vi "Guys Version_Acquire Pack and Push.vi"(9 "FIFO Refs":T1={"FIFO 0"="Simulation FIFO 0", "FIFO 1"="Simulation FIFO 1", "FIFO 2"="Simulation FIFO 2", "FIFO 3"="Simulation FIFO 3", "FIFO 4"="Simulation FIFO 4", "FIFO 5"="Simulation FIFO 5"}, 11 "Input Valid":bool) -> (3 "Ready for Input":bool)   [LabVIEW 2014]
uses:
  FPGA_Controls/Acquisition FIFOs Cluster.ctl
  <vilib>/rvi/eio/common/nirviEmuTemplateMethod_errors.vi
  <vilib>/rvi/DataTransferAndStorage/Container/Common/niFpgaContainerExecOnDevCompGetState.vi
  <vilib>/rvi/Emulation/niFpgaEmulationIsFPGAContextNoSignature.vi
  <vilib>/rvi/Emulation/niFpgaSctlEmulationGetInTimedLoop.vi
  <vilib>/rvi/errors/niFpgaSetErrorForExecOnDevCompSimple.vi
  <vilib>/rvi/eio/common/nirviEmuReportErrorAndStop.vi
  <vilib>/rvi/DataTransferAndStorage/Container/Common/niFpgaContainerGetUniqueNameForEmu.vi
  <vilib>/rvi/FIFO/Fifo_Resource/nirvififoEmulationSetSize.vi
  <vilib>/rvi/FIFO/Fifo_Resource/nirviFifoEmulationQueueMgr.vi
  <instcachedir>/0/nirviFifoEmulationQueueMgr_E5CAEC123FF24DC58D834DCA3CDAA9B5.lvgen/nirviFifoEmulationQueueMgr_E5CAEC123FF24DC58D834DCA3CDAA9B5_016.vi
  <vilib>/rvi/FIFO/Fifo_Resource/nirvififoEmulationDetermineInputValidOut.vi
  <vilib>/rvi/FIFO/Fifo_Resource/nirvififoEmulationCreateLock.vi
  <vilib>/rvi/Emulation/niFpgaProcessEmulError.vi
  <vilib>/rvi/FIFO/Fifo_Resource/nirvififoEmulationObtainLock.vi
  <vilib>/rvi/FIFO/Fifo_Resource/nirvififoEmulationReleaseLock.vi
  <vilib>/rvi/occurrence/nirviWaitOnOccurrenceBase.vi
  <vilib>/rvi/errors/nirviReportUnexpectedCaseInternalError.vi
  <vilib>/rvi/errors/nirviReportUnexpectedCaseInternalError (U32).vi
  <vilib>/rvi/interface/RandomDataEmulation/niFpgaRandomDataHandleErrors.vi
  <vilib>/eio/EIONode/EIONode.xnode
  <vilib>/rvi/DataTransferAndStorage/Container/XNode/niFpgaContainer.xnode
  <vilib>/rvi/FIFO/Fifo_Resource/niFpgaFifoEmulationRefIn.vi
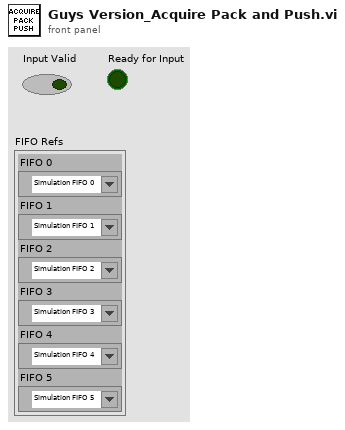
[diagram p1: front panel]
types:
  T1 = typedef "Acquisition FIFOs Cluster.ctl" = cluster{"FIFO 0":refnum<k21>, "FIFO 1":refnum<k21>, "FIFO 2":refnum<k21>, "FIFO 3":refnum<k21>, "FIFO 4":refnum<k21>, "FIFO 5":refnum<k21>}
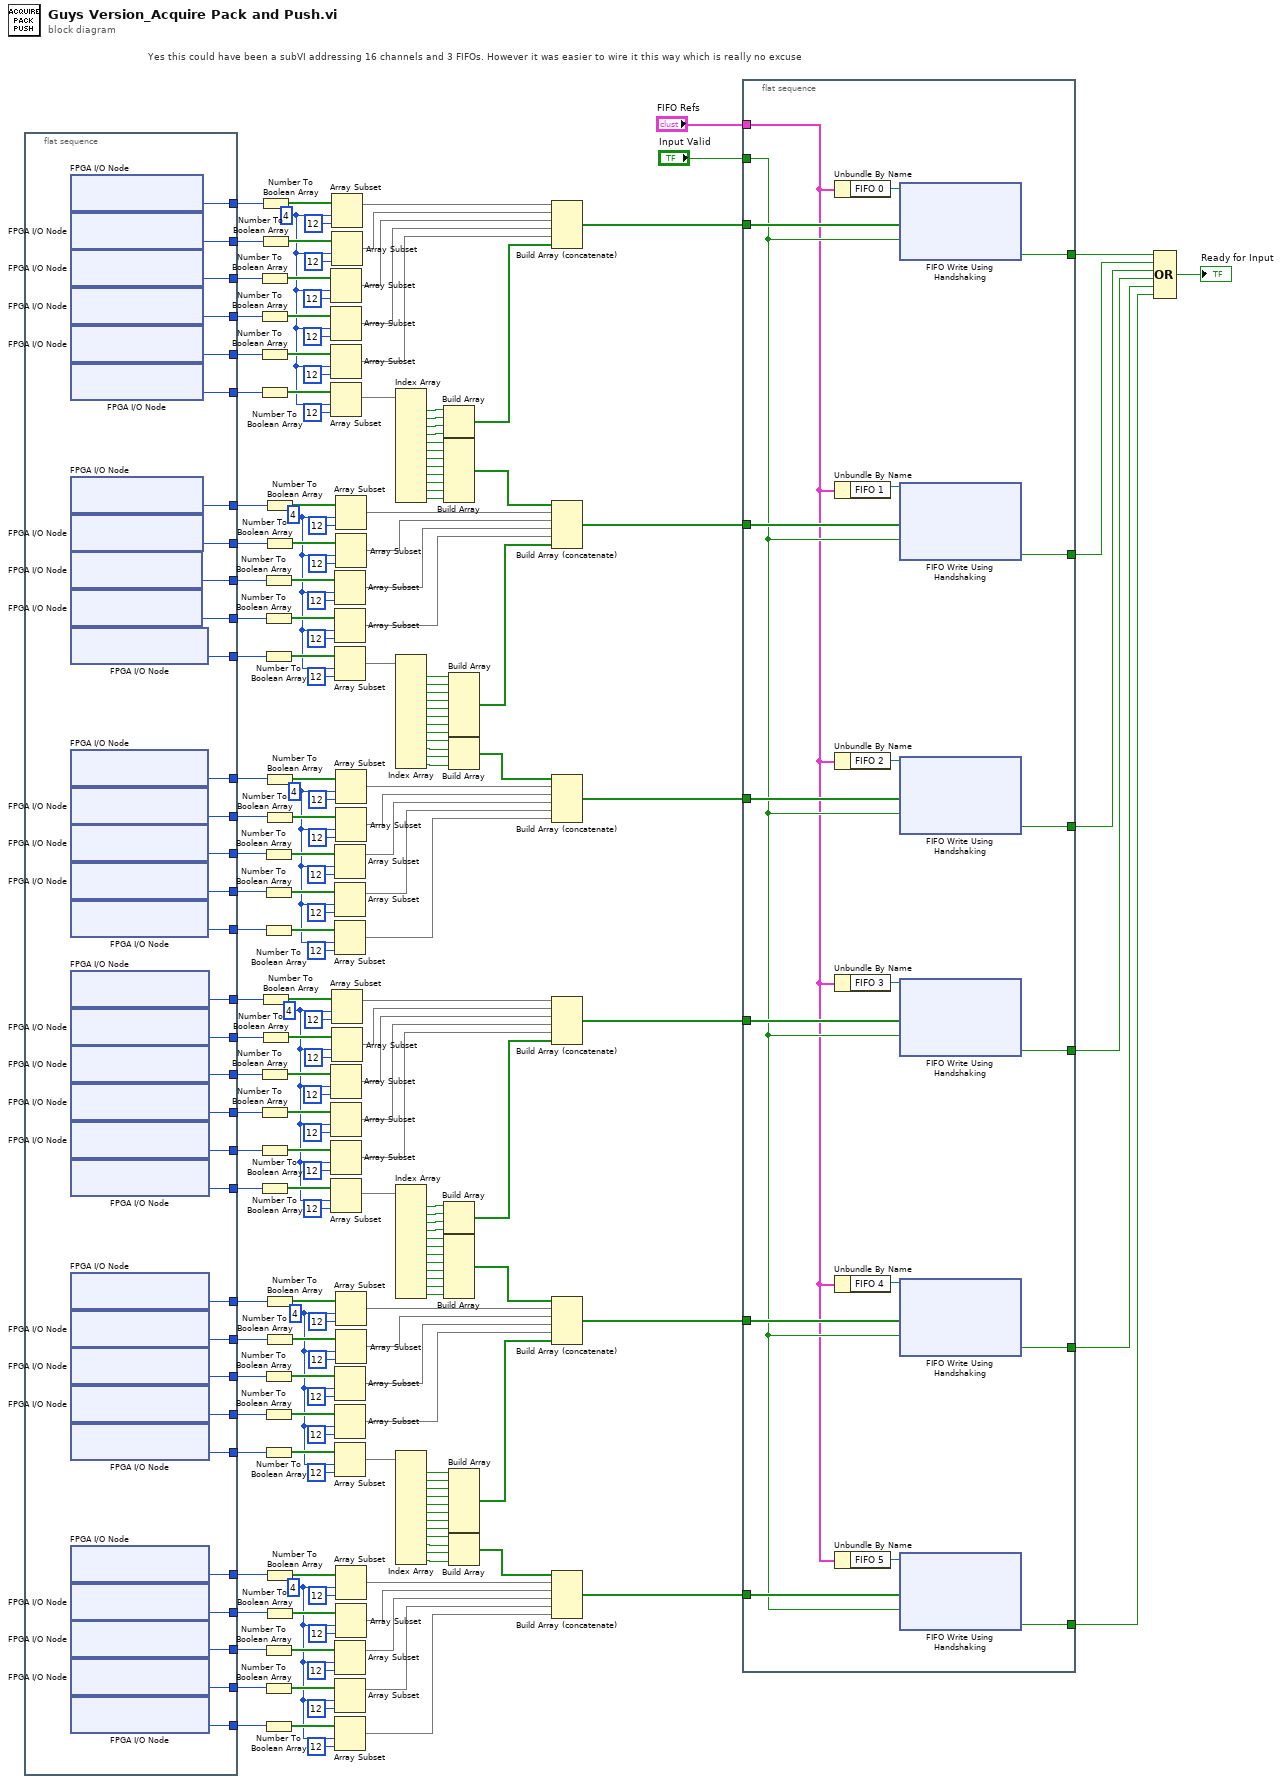
[diagram p0: block diagram]
diagram:
  w1 = 4 ("length")
  w2 = 4 ("index")
  w3 = 4 ("index")
  w4 = 4 ("index")
  w5 = 4 ("index")
  w6 = 4 ("index")
  # "Yes this could have been a subVI addressing 16 channels and 3 FIFOs. However it was easier to wire it this way which is really no excuse"
  n1 = flat-sequence {
    tunnel: [w237] -> w86
    tunnel: [w236] -> w87
    tunnel: [w235] -> w88
    tunnel: [w234] -> w89
    tunnel: [w233] -> w90
    tunnel: [w232] -> w91
    tunnel: [w231] -> w92
    tunnel: [w230] -> w93
    tunnel: [w229] -> w94
    tunnel: [w228] -> w95
    tunnel: [w227] -> w96
    tunnel: [w226] -> w97
    tunnel: [w225] -> w98
    tunnel: [w224] -> w99
    tunnel: [w223] -> w100
    tunnel: [w222] -> w101
    tunnel: [w221] -> w108
    tunnel: [w220] -> w109
    tunnel: [w219] -> w110
    tunnel: [w218] -> w111
    tunnel: [w217] -> w112
    tunnel: [w216] -> w113
    tunnel: [w215] -> w114
    tunnel: [w214] -> w115
    tunnel: [w213] -> w116
    tunnel: [w212] -> w117
    tunnel: [w211] -> w118
    tunnel: [w210] -> w119
    tunnel: [w209] -> w120
    tunnel: [w208] -> w121
    tunnel: [w207] -> w122
    tunnel: [w206] -> w123
    frame #0 {
      n2 = xnode "FPGA I/O Node"() -> ("IO Module\\AI A0"=w237:i16)  [unwired: 1 in, 1 out]
      n3 = xnode "FPGA I/O Node"() -> ("IO Module\\AI A1"=w236:i16)  [unwired: 1 in, 1 out]
      n4 = xnode "FPGA I/O Node"() -> ("IO Module\\AI A2"=w235:i16)  [unwired: 1 in, 1 out]
      n5 = xnode "FPGA I/O Node"() -> ("IO Module\\AI A3"=w234:i16)  [unwired: 1 in, 1 out]
      n6 = xnode "FPGA I/O Node"() -> ("IO Module\\AI A4"=w233:i16)  [unwired: 1 in, 1 out]
      n7 = xnode "FPGA I/O Node"() -> ("IO Module\\AI A5"=w232:i16)  [unwired: 1 in, 1 out]
      n8 = xnode "FPGA I/O Node"() -> ("IO Module\\AI A6"=w231:i16)  [unwired: 1 in, 1 out]
      n9 = xnode "FPGA I/O Node"() -> ("IO Module\\AI A7"=w230:i16)  [unwired: 1 in, 1 out]
      n10 = xnode "FPGA I/O Node"() -> ("IO Module\\AI B8"=w229:i16)  [unwired: 1 in, 1 out]
      n11 = xnode "FPGA I/O Node"() -> ("IO Module\\AI B9"=w228:i16)  [unwired: 1 in, 1 out]
      n12 = xnode "FPGA I/O Node"() -> ("IO Module\\AI B10"=w227:i16)  [unwired: 1 in, 1 out]
      n13 = xnode "FPGA I/O Node"() -> ("IO Module\\AI B11"=w226:i16)  [unwired: 1 in, 1 out]
      n14 = xnode "FPGA I/O Node"() -> ("IO Module\\AI B12"=w225:i16)  [unwired: 1 in, 1 out]
      n15 = xnode "FPGA I/O Node"() -> ("IO Module\\AI B13"=w224:i16)  [unwired: 1 in, 1 out]
      n16 = xnode "FPGA I/O Node"() -> ("IO Module\\AI B14"=w223:i16)  [unwired: 1 in, 1 out]
      n17 = xnode "FPGA I/O Node"() -> ("IO Module\\AI B15"=w222:i16)  [unwired: 1 in, 1 out]
      n18 = xnode "FPGA I/O Node"() -> ("IO Module\\AI C16"=w206:i16)  [unwired: 1 in, 1 out]
      n19 = xnode "FPGA I/O Node"() -> ("IO Module\\AI C17"=w207:i16)  [unwired: 1 in, 1 out]
      n20 = xnode "FPGA I/O Node"() -> ("IO Module\\AI C18"=w208:i16)  [unwired: 1 in, 1 out]
      n21 = xnode "FPGA I/O Node"() -> ("IO Module\\AI C19"=w209:i16)  [unwired: 1 in, 1 out]
      n22 = xnode "FPGA I/O Node"() -> ("IO Module\\AI C20"=w210:i16)  [unwired: 1 in, 1 out]
      n23 = xnode "FPGA I/O Node"() -> ("IO Module\\AI C21"=w211:i16)  [unwired: 1 in, 1 out]
      n24 = xnode "FPGA I/O Node"() -> ("IO Module\\AI C22"=w212:i16)  [unwired: 1 in, 1 out]
      n25 = xnode "FPGA I/O Node"() -> ("IO Module\\AI C23"=w213:i16)  [unwired: 1 in, 1 out]
      n26 = xnode "FPGA I/O Node"() -> ("IO Module\\AI D24"=w214:i16)  [unwired: 1 in, 1 out]
      n27 = xnode "FPGA I/O Node"() -> ("IO Module\\AI D25"=w215:i16)  [unwired: 1 in, 1 out]
      n28 = xnode "FPGA I/O Node"() -> ("IO Module\\AI D26"=w216:i16)  [unwired: 1 in, 1 out]
      n29 = xnode "FPGA I/O Node"() -> ("IO Module\\AI D27"=w217:i16)  [unwired: 1 in, 1 out]
      n30 = xnode "FPGA I/O Node"() -> ("IO Module\\AI D28"=w218:i16)  [unwired: 1 in, 1 out]
      n31 = xnode "FPGA I/O Node"() -> ("IO Module\\AI D29"=w219:i16)  [unwired: 1 in, 1 out]
      n32 = xnode "FPGA I/O Node"() -> ("IO Module\\AI D30"=w220:i16)  [unwired: 1 in, 1 out]
      n33 = xnode "FPGA I/O Node"() -> ("IO Module\\AI D31"=w221:i16)  [unwired: 1 in, 1 out]
    }
  }
  n34 = Number To Boolean Array(number=w88) -> (Boolean array=w19:bool[])
  n35 = Number To Boolean Array(number=w89) -> (Boolean array=w16:bool[])
  n36 = Number To Boolean Array(number=w90) -> (Boolean array=w25:bool[])
  n37 = Number To Boolean Array(number=w91) -> (Boolean array=w22:bool[])
  n38 = Number To Boolean Array(number=w121) -> (Boolean array=w190:bool[])
  n39 = Number To Boolean Array(number=w120) -> (Boolean array=w193:bool[])
  n40 = Number To Boolean Array(number=w119) -> (Boolean array=w184:bool[])
  n41 = Number To Boolean Array(number=w118) -> (Boolean array=w187:bool[])
  n42 = Number To Boolean Array(number=w86) -> (Boolean array=w10:bool[])
  n43 = Number To Boolean Array(number=w87) -> (Boolean array=w13:bool[])
  n44 = Number To Boolean Array(number=w123) -> (Boolean array=w199:bool[])
  n45 = Number To Boolean Array(number=w122) -> (Boolean array=w196:bool[])
  n46 = Number To Boolean Array(number=w94) -> (Boolean array=w43:bool[])
  n47 = Number To Boolean Array(number=w95) -> (Boolean array=w46:bool[])
  n48 = Number To Boolean Array(number=w96) -> (Boolean array=w41:bool[])
  n49 = Number To Boolean Array(number=w99) -> (Boolean array=w77:bool[])
  n50 = Number To Boolean Array(number=w100) -> (Boolean array=w74:bool[])
  n51 = Number To Boolean Array(number=w101) -> (Boolean array=w79:bool[])
  n52 = Number To Boolean Array(number=w115) -> (Boolean array=w166:bool[])
  n53 = Number To Boolean Array(number=w114) -> (Boolean array=w163:bool[])
  n54 = Number To Boolean Array(number=w113) -> (Boolean array=w168:bool[])
  n55 = Number To Boolean Array(number=w110) -> (Boolean array=w132:bool[])
  n56 = Number To Boolean Array(number=w109) -> (Boolean array=w135:bool[])
  n57 = Number To Boolean Array(number=w108) -> (Boolean array=w130:bool[])
  n58 = Number To Boolean Array(number=w92) -> (Boolean array=w50:bool[])
  n59 = Number To Boolean Array(number=w93) -> (Boolean array=w47:bool[])
  n60 = Number To Boolean Array(number=w97) -> (Boolean array=w70:bool[])
  n61 = Number To Boolean Array(number=w98) -> (Boolean array=w73:bool[])
  n62 = Number To Boolean Array(number=w117) -> (Boolean array=w159:bool[])
  n63 = Number To Boolean Array(number=w116) -> (Boolean array=w162:bool[])
  n64 = Number To Boolean Array(number=w112) -> (Boolean array=w139:bool[])
  n65 = Number To Boolean Array(number=w111) -> (Boolean array=w136:bool[])
  n66 = Array Subset(array=w19, index=w6, length=12) -> (w20:bool[])
  n67 = Array Subset(array=w16, index=w6, length=12) -> (w21:bool[])
  n68 = Array Subset(array=w25, index=w6, length=12) -> (w26:bool[])
  n69 = Array Subset(array=w22, index=w6, length=12) -> (w27:bool[])
  n70 = Array Subset(array=w190, index=w3, length=12) -> (w189:bool[])
  n71 = Array Subset(array=w193, index=w3, length=12) -> (w188:bool[])
  n72 = Array Subset(array=w184, index=w3, length=12) -> (w183:bool[])
  n73 = Array Subset(array=w187, index=w3, length=12) -> (w182:bool[])
  n74 = Array Subset(array=w10, index=w6, length=12) -> (w14:bool[])
  n75 = Array Subset(array=w13, index=w6, length=12) -> (w15:bool[])
  n76 = Array Subset(array=w199, index=w3, length=12) -> (w195:bool[])
  n77 = Array Subset(array=w196, index=w3, length=12) -> (w194:bool[])
  n78 = Array Subset(array=w43, index=w5, length=12) -> (w54:bool[])
  n79 = Array Subset(array=w46, index=w5, length=12) -> (w55:bool[])
  n80 = Array Subset(array=w41, index=w5, length=12) -> (w56:bool[])
  n81 = Array Subset(array=w77, index=w4, length=12) -> (w83:bool[])
  n82 = Array Subset(array=w74, index=w4, length=12) -> (w84:bool[])
  n83 = Array Subset(array=w79, index=w4, length=12) -> (w85:bool[])
  n84 = Array Subset(array=w166, index=w2, length=12) -> (w155:bool[])
  n85 = Array Subset(array=w163, index=w2, length=12) -> (w154:bool[])
  n86 = Array Subset(array=w168, index=w2, length=12) -> (w153:bool[])
  n87 = Array Subset(array=w132, index=w1, length=12) -> (w126:bool[])
  n88 = Array Subset(array=w135, index=w1, length=12) -> (w125:bool[])
  n89 = Array Subset(array=w130, index=w1, length=12) -> (w124:bool[])
  n90 = Array Subset(array=w50, index=w5, length=12) -> (w52:bool[])
  n91 = Array Subset(array=w47, index=w5, length=12) -> (w53:bool[])
  n92 = Array Subset(array=w70, index=w4, length=12) -> (w81:bool[])
  n93 = Array Subset(array=w73, index=w4, length=12) -> (w82:bool[])
  n94 = Array Subset(array=w159, index=w2, length=12) -> (w157:bool[])
  n95 = Array Subset(array=w162, index=w2, length=12) -> (w156:bool[])
  n96 = Array Subset(array=w139, index=w1, length=12) -> (w128:bool[])
  n97 = Array Subset(array=w136, index=w1, length=12) -> (w127:bool[])
  n98 = Index Array(array=w27) -> (element #1=w28:bool, element #2=w29:bool, element #3=w30:bool, element #4=w31:bool, element #5=w33:bool, element #6=w34:bool, element #7=w35:bool, element #8=w36:bool, element #9=w37:bool, element #10=w38:bool, element #11=w39:bool, element #12=w40:bool)  [unwired: 12 in]
  n99 = Index Array(array=w56) -> (element #1=w57:bool, element #2=w58:bool, element #3=w59:bool, element #4=w60:bool, element #5=w61:bool, element #6=w62:bool, element #7=w63:bool, element #8=w64:bool, element #9=w66:bool, element #10=w67:bool, element #11=w68:bool, element #12=w69:bool)  [unwired: 12 in]
  n100 = Index Array(array=w182) -> (element #1=w181:bool, element #2=w180:bool, element #3=w179:bool, element #4=w178:bool, element #5=w176:bool, element #6=w175:bool, element #7=w174:bool, element #8=w173:bool, element #9=w172:bool, element #10=w171:bool, element #11=w170:bool, element #12=w169:bool)  [unwired: 12 in]
  n101 = Index Array(array=w153) -> (element #1=w152:bool, element #2=w151:bool, element #3=w150:bool, element #4=w149:bool, element #5=w148:bool, element #6=w147:bool, element #7=w146:bool, element #8=w145:bool, element #9=w143:bool, element #10=w142:bool, element #11=w141:bool, element #12=w140:bool)  [unwired: 12 in]
  n102 = Build Array(w28, w29, w30, w31) -> (w32:bool[])
  n103 = Build Array(w33, w34, w35, w36, w37, w38, w39, w40) -> (w51:bool[])
  n104 = Build Array(w181, w180, w179, w178) -> (w177:bool[])
  n105 = Build Array(w176, w175, w174, w173, w172, w171, w170, w169) -> (w158:bool[])
  n106 = Build Array(w57, w58, w59, w60, w61, w62, w63, w64) -> (w65:bool[])
  n107 = Build Array(w66, w67, w68, w69) -> (w80:bool[])
  n108 = Build Array(w152, w151, w150, w149, w148, w147, w146, w145) -> (w144:bool[])
  n109 = Build Array(w143, w142, w141, w140) -> (w129:bool[])
  n110 = Build Array (concatenate)(w14, w15, w20, w21, w26, w32) -> (w102:bool[])
  n111 = Build Array (concatenate)(w51, w52, w53, w54, w55, w65) -> (w103:bool[])
  n112 = Build Array (concatenate)(w80, w81, w82, w83, w84, w85) -> (w104:bool[])
  n113 = Build Array (concatenate)(w195, w194, w189, w188, w183, w177) -> (w107:bool[])
  n114 = Build Array (concatenate)(w158, w157, w156, w155, w154, w144) -> (w106:bool[])
  n115 = Build Array (concatenate)(w129, w128, w127, w126, w125, w124) -> (w105:bool[])
  n116 = flat-sequence {
    tunnel: w102 -> [w257]
    tunnel: w103 -> [w256]
    tunnel: w104 -> [w255]
    tunnel: w105 -> [w254]
    tunnel: w106 -> [w253]
    tunnel: w107 -> [w252]
    tunnel: [w251] -> w200
    tunnel: [w250] -> w201
    tunnel: [w249] -> w202
    tunnel: [w248] -> w203
    tunnel: [w247] -> w204
    tunnel: [w246] -> w205
    tunnel: "Input Valid" -> [w245]
    tunnel: "FIFO Refs" -> [w238]
    frame #0 {
      n117 = Unbundle By Name(w238) -> ("FIFO 0"=w244:refnum<k21>)
      n118 = Unbundle By Name(w238) -> ("FIFO 1"=w243:refnum<k21>)
      n119 = Unbundle By Name(w238) -> ("FIFO 2"=w242:refnum<k21>)
      n120 = Unbundle By Name(w238) -> ("FIFO 3"=w241:refnum<k21>)
      n121 = Unbundle By Name(w238) -> ("FIFO 4"=w240:refnum<k21>)
      n122 = Unbundle By Name(w238) -> ("FIFO 5"=w239:refnum<k21>)
      n123 = xnode ("FIFO Write Using Handshaking")("Element"=w257, "Input Valid"=w245, "FIFO In"=w244) -> ("Ready for Input"=w251:bool)  [unwired: 1 out]
      n124 = xnode ("FIFO Write Using Handshaking")("Element"=w256, "Input Valid"=w245, "FIFO In"=w243) -> ("Ready for Input"=w250:bool)  [unwired: 1 out]
      n125 = xnode ("FIFO Write Using Handshaking")("Element"=w255, "Input Valid"=w245, "FIFO In"=w242) -> ("Ready for Input"=w249:bool)  [unwired: 1 out]
      n126 = xnode ("FIFO Write Using Handshaking")("Element"=w252, "Input Valid"=w245, "FIFO In"=w241) -> ("Ready for Input"=w248:bool)  [unwired: 1 out]
      n127 = xnode ("FIFO Write Using Handshaking")("Element"=w253, "Input Valid"=w245, "FIFO In"=w240) -> ("Ready for Input"=w247:bool)  [unwired: 1 out]
      n128 = xnode ("FIFO Write Using Handshaking")("Element"=w254, "Input Valid"=w245, "FIFO In"=w239) -> ("Ready for Input"=w246:bool)  [unwired: 1 out]
    }
  }
  n129 = Compound Arithmetic op=OR(w200, w201, w202, w203, w204, w205) -> (→"Ready for Input":bool)
